vi "AlliGator Check Decay Pre-Processing Steps Needed.vi"(10 "Decay Preprocessing Parameters":T1={"Background Subtraction"=FALSE, "Straighten Decay"=FALSE, "Reverse Gates"=FALSE, "1-Normalized Decay"=FALSE, "Smoothen Decay"=FALSE, "Smoothing Parameter"=0.0, "Shift Decay"=FALSE, "Decay Shift Parameters"={"Type"=enum."Default", "Shift"=0.0, "Threshold"=0.0, "Rotate"=FALSE}, "Extrapolate Decay"=FALSE, "Additional Points"=0, "Head Fraction"=0.0, "Pixel-Normalize Decay"=FALSE, "Use Periodicity"=FALSE, "Use Cursors"=FALSE, "Tail Fraction"=0.0, "Use Decay Pre-Processing"=FALSE, "Fold Decay"=FALSE, "# Folds"=1, "[0-1]-Normalized Decay"=FALSE} {"# Folds" min=1}, 11 "Preprocessing Steps Order in":string[](array[string])) -> (1 "Preprocessing needed?":bool, 2 "Decay Preprocessing Parameters (dup)":T1={"Background Subtraction"=FALSE, "Straighten Decay"=FALSE, "Reverse Gates"=FALSE, "1-Normalized Decay"=FALSE, "Smoothen Decay"=FALSE, "Smoothing Parameter"=0.0, "Shift Decay"=FALSE, "Decay Shift Parameters"={"Type"=enum."Default", "Shift"=0.0, "Threshold"=0.0, "Rotate"=FALSE}, "Extrapolate Decay"=FALSE, "Additional Points"=0, "Head Fraction"=0.0, "Pixel-Normalize Decay"=FALSE, "Use Periodicity"=FALSE, "Use Cursors"=FALSE, "Tail Fraction"=0.0, "Use Decay Pre-Processing"=FALSE, "Fold Decay"=FALSE, "# Folds"=1, "[0-1]-Normalized Decay"=FALSE} {"# Folds" min=1}, 3 "Preprocessing Steps Order out":string[](array[string]))   [LabVIEW 2021, in "AlliGator Phasor Plot.lvlib"]
doc: "Checks whether any decay pre-processing is needed."
uses:
  AlliGator Phasor Plot.lvlib
  AlliGator Decay Preprocessing Parameters.ctl
  Graphs/XY Graph/XY Graph Plot Shift Parameters.ctl
  Graphs/XY Graph/XY Graph Plot Shift Method.ctl
  Graphs/XY Graph/XY Graph Add-Ons.lvlib
  AlliGator Decay Preprocessing.lvlib
panel:
  # "see the AlliGator License on the block diagram (Ctrl+E or Window:Show Block Diagram)"
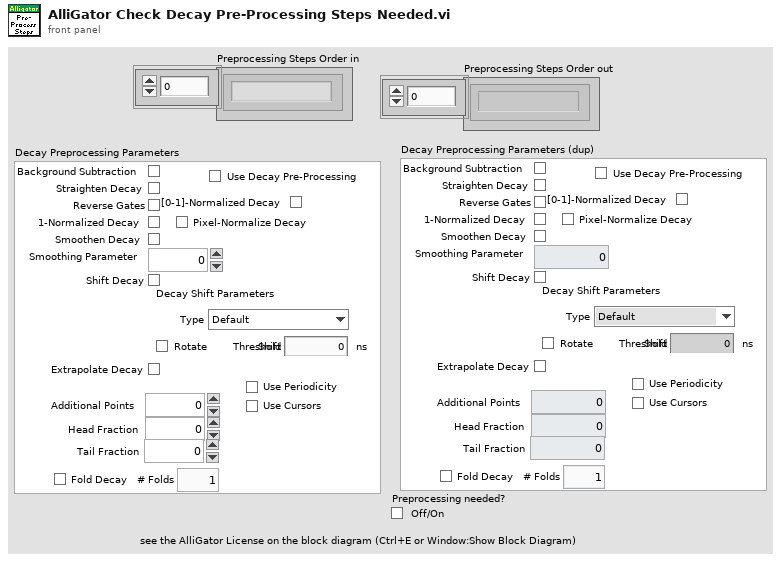
[diagram p1: front panel]
types:
  T1 = typedef "AlliGator Decay Analysis.lvlib/AlliGator Decay Preprocessing.lvlib/AlliGator Decay Preprocessing Parameters.ctl" = cluster{"Background Subtraction":bool, "Straighten Decay":bool, "Reverse Gates":bool, "1-Normalized Decay":bool, "Smoothen Decay":bool, "Smoothing Parameter":dbl, "Shift Decay":bool, "Decay Shift Parameters":T2, "Extrapolate Decay":bool, "Additional Points":u32, "Head Fraction":dbl, "Pixel-Normalize Decay":bool, "Use Periodicity":bool, "Use Cursors":bool, "Tail Fraction":dbl, "Use Decay Pre-Processing":bool, "Fold Decay":bool, "# Folds":u32, "[0-1]-Normalized Decay":bool}
  T2 = typedef "XY Graph Add-Ons.lvlib/XY Graph Plot Shift Parameters.ctl" = cluster{"Type":T3, "Shift":dbl[unit], "Threshold":dbl, "Rotate":bool}
  T3 = typedef "XY Graph Add-Ons.lvlib/XY Graph Plot Shift Method.ctl" = enum16{"Default", "CFD", "Threshold", "Cross-Correlation"}
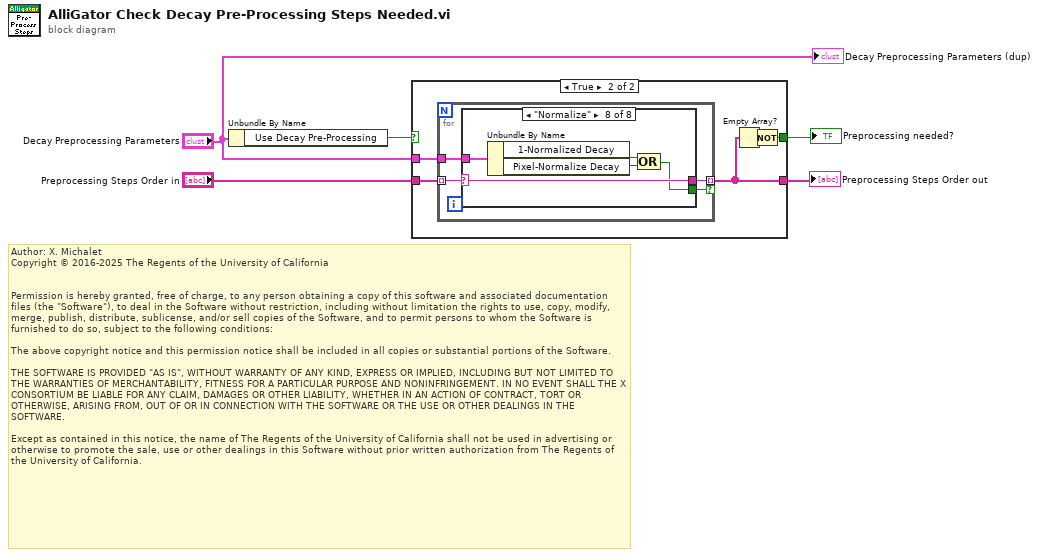
[diagram p0: block diagram]
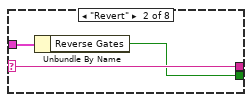
[diagram p4: hidden frame]
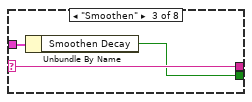
[diagram p5: hidden frame]
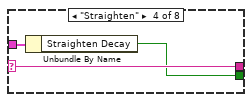
[diagram p6: hidden frame]
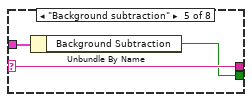
[diagram p7: hidden frame]
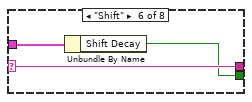
[diagram p8: hidden frame]
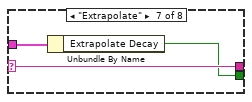
[diagram p9: hidden frame]
diagram:
  # "Author: X. Michalet\nCopyright © 2016-2025 The Regents of the University of California\n \n\nPermission is hereby granted, free of charge, to any person obtaining a copy of this software and associated documentation files (the \"Software\"), to deal in the Software without restriction, including without limitation the rights to use, copy, modify, merge, publish, distribute, sublicense, and/or sell copies of the Software, and to permit persons to whom the Software is furnished to do so, subject to the following conditions:\n\nThe above copyright notice and this permission notice shall be included in all copies or substantial portions of the Software.\n\nTHE SOFTWARE IS PROVIDED \"AS IS\", WITHOUT WARRANTY OF ANY KIND, EXPRESS OR IMPLIED, INCLUDING BUT NOT LIMITED TO THE WARRANTIES OF MERCHANTABILITY, FITNESS FOR A PARTICULAR PURPOSE AND NONINFRINGEMENT. IN NO EVENT SHALL THE X CONSORTIUM BE LIABLE FOR ANY CLAIM, DAMAGES OR OTHER LIABILITY, WHETHER IN AN ACTION OF CONTRACT, TORT OR OTHERWISE, ARISING FROM, OUT OF OR IN CONNECTION WITH THE SOFTWARE OR THE USE OR OTHER DEALINGS IN THE SOFTWARE.\n\nExcept as contained in this notice, the name of The Regents of the University of California shall not be used in advertising or otherwise to promote the sale, use or other dealings in this Software without prior written authorization from The Regents of the University of California."
  n1 = Unbundle By Name("Decay Preprocessing Parameters") -> ("Use Decay Pre-Processing"=w5:bool)
  n2 = case shown="True" w5 {
    selector: w5 -> [w7 _]
    tunnel: [w7 w8] -> w4
    tunnel: "Preprocessing Steps Order in" -> [w6 w12]
    tunnel: "Decay Preprocessing Parameters" -> [_ w11]
    tunnel: [w6 w10] -> w2
    frame False {
    }
    frame True {
      n3 = for {
        tunnel: w12 -> [w16] mode=indexing
        tunnel: w11 -> [w15]
        tunnel: [w14] -> w10 mode=indexing if=w13
        n4 = case shown="\"Normalize\"" w16 {
          selector: w16 -> [_ w18 w21 w24 w27 w30 w33 w38]
          tunnel: w15 -> [_ w19 w22 w25 w28 w31 w34 w39]
          tunnel: [_ w18 w21 w24 w27 w30 w33 w38] -> w14
          tunnel: [_ w17 w20 w23 w26 w29 w32 w36] -> w13
          frame "", Default {
          }
          frame "Revert" {
            n5 = Unbundle By Name(w19) -> ("Reverse Gates"=w17:bool)
          }
          frame "Smoothen" {
            n6 = Unbundle By Name(w22) -> ("Smoothen Decay"=w20:bool)
          }
          frame "Straighten" {
            n7 = Unbundle By Name(w25) -> ("Straighten Decay"=w23:bool)
          }
          frame "Background subtraction" {
            n8 = Unbundle By Name(w28) -> ("Background Subtraction"=w26:bool)
          }
          frame "Shift" {
            n9 = Unbundle By Name(w31) -> ("Shift Decay"=w29:bool)
          }
          frame "Extrapolate" {
            n10 = Unbundle By Name(w34) -> ("Extrapolate Decay"=w32:bool)
          }
          frame "Normalize" {
            n11 = Unbundle By Name(w39) -> ("1-Normalized Decay"=w37:bool, "Pixel-Normalize Decay"=w35:bool)
            n12 = Compound Arithmetic op=OR(w37, w35) -> (w36:bool)
          }
        }
      }
      n13 = Empty Array?(array=w10) -> (empty?=w9:bool)
      n14 = Not(x=w9) -> (.not. x?=w8:bool)
    }
  }
  "Preprocessing needed?" <- w4
  "Preprocessing Steps Order out" <- w2
  "Decay Preprocessing Parameters (dup)" <- "Decay Preprocessing Parameters"
